vi "Insert View into Subpanel.vi"(0 "GUI Container Actor in":refnum<class "GUI Container Actor.lvclass">, 5 "View":string, 7 "View Hierarchy Level":i32, 9 "Subpanel":string, 11 "error in (no error)":errorcluster) -> (4 "GUI Container Actor out":refnum<class "GUI Container Actor.lvclass">, 15 "error out":errorcluster)   [LabVIEW 2017, in "GUI Views.lvlib" / "GUI Container Actor.lvclass"]
doc: "Inserts the Front Panel of a specified Actor Core VI of the the specified View class hierarchy into a specified subpanel\n\n<b> View </b> String theat contains the name of the View\n\n<b> View Hierarchy Level</b> the level on the subclassing hierarchy of the GUI View actor, it is used to choose the Actor Core Front Panel among all the exisiting sublcasses of the GUI VIew Actor present in the View specified above\n\n<b>Subpanel</b> string designating in which subpanel the Front Panel specified in the above terminals has to be inserted"
uses:
  GUI Container Actor.lvclass
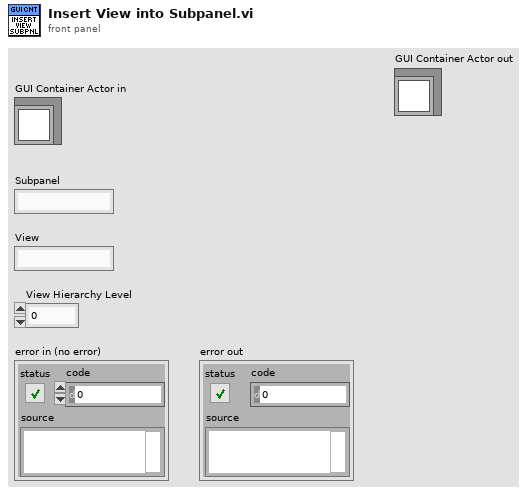
[diagram p1: front panel]
types:
  T1 = typedef "GUI Views.lvlib/GUI Container Actor.lvclass/View Status.ctl" = cluster{"View Details":T2, "Front Panel Statuses":T3[]}
  T2 = typedef "GUI Views.lvlib/GUI Container Actor.lvclass/View Details.ctl" = cluster{"Enqueuer":refnum<class "Message Enqueuer.lvclass">, "VI References":refnum<vi>[], "FP References":refnum<vi>[]}
  T3 = typedef "GUI Views.lvlib/GUI Container Actor.lvclass/FP Status.ctl" = cluster{"FP Open":bool, "Inserted in Subpanel":bool, "Subpanel":string}
  T4 = typedef "GUI Views.lvlib/GUI Container Actor.lvclass/VI References.ctl" = cluster{"FP Ref":refnum<vi>, "VI Ref":refnum<vi>}
  T5 = typedef "GUI Views.lvlib/GUI Container Actor.lvclass/Subpanel Status.ctl" = cluster{"Subpanel Ref":refnum<vi>, "Inserted View":string, "Inserted View Hierarchy Level":i32}
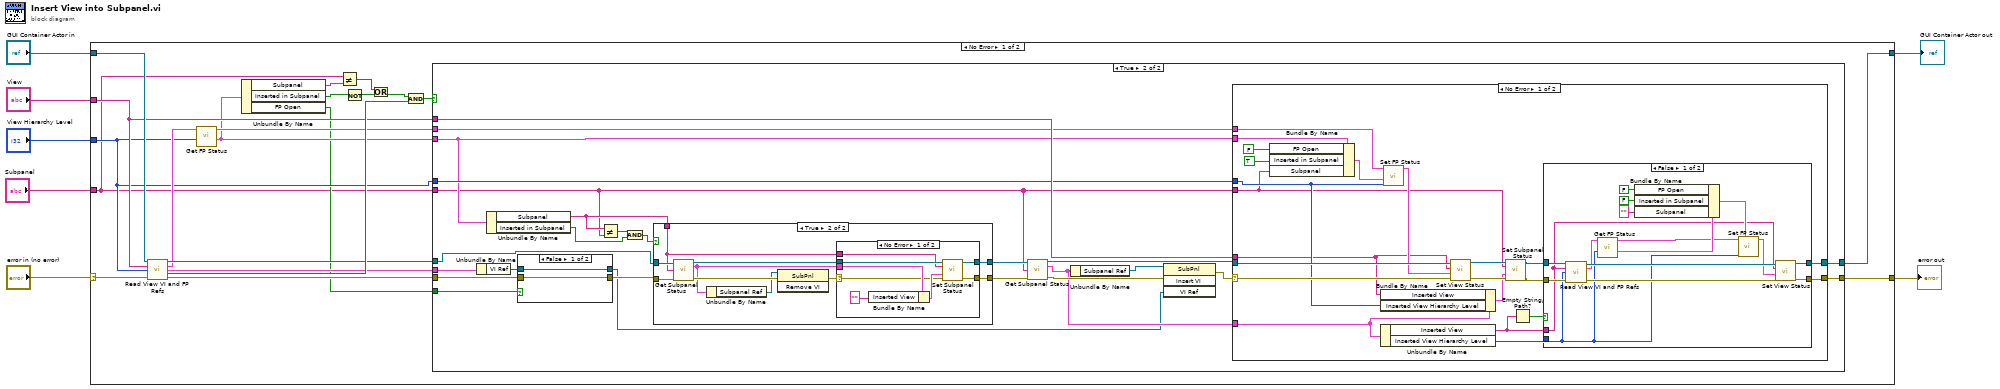
[diagram p0: block diagram]
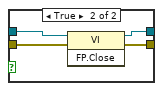
[diagram p7: hidden frame]
diagram:
  n1 = case shown="No Error" "error in (no error)" {
    selector: "error in (no error)" -> [w27 w126]
    tunnel: [w28 w126] -> w7
    tunnel: "GUI Container Actor in" -> [w26 w127]
    tunnel: "Subpanel" -> [w10 _]
    tunnel: "View Hierarchy Level" -> [w15 _]
    tunnel: "View" -> [w20 _]
    tunnel: [w19 w127] -> w1
    frame No Error {
      n2 = call "Read View VI and FP Refs.vi"("GUI Container Actor in"=w26, "View"=w20, "View Hierarchy Level"=w15, "error in (no error)"=w27) -> ("GUI Container Actor out"=w22:refnum<class "GUI Container Actor.lvclass">, "View Status"=w18:T1, "VI References"=w21:T4, "View Found"=w25:bool, "error out"=w23:errorcluster)  [unwired: 7 in]
      n3 = call "Get FP Status.vi"("View Hierarchy Level"=w15, "View Status in"=w18) -> ("FP Status"=w16:T3, "View Status out"=w17:T1)  [unwired: 8 in]
      n4 = Unbundle By Name(w16) -> ("Subpanel"=w13:string, "Inserted in Subpanel"=w11:bool, "FP Open"=w14:bool)
      n5 = Not Equal?(x=w10, y=w13) -> (x != y?=w8:bool)
      n6 = Not(x=w11) -> (.not. x?=w12:bool)
      n7 = Or(x=w8, y=w12) -> (x .or. y?=w9:bool)
      n8 = Compound Arithmetic op=AND(w9, w25) -> (w24:bool)
      n9 = case shown="True" w24 {
        tunnel: [w30 w49] -> w28
        tunnel: w10 -> [_ w31]
        tunnel: w23 -> [w30 w52]
        tunnel: w22 -> [w29 w35]
        tunnel: w21 -> [_ w54]
        tunnel: w14 -> [_ w51]
        tunnel: w20 -> [_ w47]
        tunnel: [w29 w46] -> w19
        tunnel: w17 -> [_ w45]
        tunnel: w16 -> [_ w33]
        tunnel: w15 -> [_ w44]
        frame False {
        }
        frame True {
          n10 = Unbundle By Name(w54) -> ("VI Ref"=w53:refnum<vi>)
          n11 = Unbundle By Name(w33) -> ("Subpanel"=w38:string, "Inserted in Subpanel"=w41:bool)
          n12 = case shown="False" w51 {
            tunnel: w53 -> [w121 w125]
            tunnel: w52 -> [w120 w124]
            tunnel: [w120 w123] -> w36
            tunnel: [w121 w122] -> w32
            frame False {
            }
            frame True {
              n13 = invoke class="VI" method="FP.Close"(reference=w125, error in=w124) -> (reference out=w122:refnum<vi>, error out=w123:errorcluster)  [unwired: 1 in, 1 out]
            }
          }
          n14 = Not Equal?(x=w38, y=w31) -> (x != y?=w39:bool)
          n15 = And(x=w39, y=w41) -> (x .and. y?=w40:bool)
          n16 = case shown="True" w40 {
            tunnel: w36 -> [w56 w67]
            tunnel: w35 -> [w57 w66]
            tunnel: [w57 w64] -> w34
            tunnel: [w56 w63] -> w37
            tunnel: w38 -> [_ w62]
            frame False {
            }
            frame True {
              n17 = call "Get Subpanel Status.vi"("GUI Container Actor in"=w66, "Subpanel"=w62, "error in (no error)"=w67) -> ("GUI Container Actor out"=w65:refnum<class "GUI Container Actor.lvclass">, "Subpanel Status"=w60:T5, "error out"=w61:errorcluster)  [unwired: 9 in, 1 out]
              n18 = Unbundle By Name(w60) -> ("Subpanel Ref"=w59:refnum<vi>)
              n19 = invoke class="SubPnl" method="Remove VI"(reference=w59, error in=w61) -> (error out=w58:errorcluster)  [unwired: 1 in, 2 out]
              n20 = case shown="No Error" w58 {
                selector: w58 -> [w68 w76]
                tunnel: w65 -> [w74 w77]
                tunnel: [w73 w77] -> w64
                tunnel: [w72 w76] -> w63
                tunnel: w62 -> [w70 _]
                tunnel: w60 -> [w69 _]
                frame No Error {
                  n21 = Bundle By Name(cluster=w69, "Inserted View"="") -> (w75:T5)
                  n22 = call "Set Subpanel Status.vi"("GUI Container Actor in"=w74, "Subpanel"=w70, "Subpanel Status"=w75, "error in (no error)"=w68) -> ("GUI Container Actor out"=w73:refnum<class "GUI Container Actor.lvclass">, "error out"=w72:errorcluster)  [unwired: 9 in, 1 out]
                }
                frame Error {
                }
              }
            }
          }
          n23 = call "Get Subpanel Status.vi"("GUI Container Actor in"=w34, "Subpanel"=w31, "error in (no error)"=w37) -> ("GUI Container Actor out"=w48:refnum<class "GUI Container Actor.lvclass">, "Subpanel Status"=w42:T5, "error out"=w55:errorcluster)  [unwired: 9 in, 1 out]
          n24 = Unbundle By Name(w42) -> ("Subpanel Ref"=w43:refnum<vi>)
          n25 = invoke class="SubPnl" method="Insert VI"(reference=w43, error in=w55, "VI Ref"=w32) -> (error out=w50:errorcluster)  [unwired: 1 in, 3 out]
          n26 = case shown="No Error" w50 {
            selector: w50 -> [w98 w119]
            tunnel: [w79 w119] -> w49
            tunnel: w48 -> [w99 w118]
            tunnel: w47 -> [w92 _]
            tunnel: [w80 w118] -> w46
            tunnel: w33 -> [w87 _]
            tunnel: w45 -> [w96 _]
            tunnel: w44 -> [w93 _]
            tunnel: w31 -> [w86 _]
            tunnel: w42 -> [w82 _]
            frame No Error {
              n27 = Bundle By Name(cluster=w87, "FP Open"=FALSE, "Inserted in Subpanel"=TRUE ("FP Open"), "Subpanel"=w86) -> (w89:T3)
              n28 = Unbundle By Name(w82) -> ("Inserted View"=w81:string, "Inserted View Hierarchy Level"=w83:i32)
              n29 = Bundle By Name(cluster=w82, "Inserted View"=w92, "Inserted View Hierarchy Level"=w93) -> (w91:T5)
              n30 = call "Set FP Status.vi"("View Hierarchy Level"=w93, "FP Status"=w89, "View Status in"=w96) -> ("View Status out"=w95:T1)  [unwired: 8 in]
              n31 = call "Set View Status.vi"("error in (no error)"=w98, "View Status"=w95, "View"=w92, "GUI Container Actor in"=w99) -> ("error out"=w94:errorcluster, "GUI Container Actor out"=w90:refnum<class "GUI Container Actor.lvclass">)  [unwired: 5 in, 1 out]
              n32 = call "Set Subpanel Status.vi"("GUI Container Actor in"=w90, "Subpanel"=w86, "Subpanel Status"=w91, "error in (no error)"=w94) -> ("GUI Container Actor out"=w85:refnum<class "GUI Container Actor.lvclass">, "error out"=w84:errorcluster)  [unwired: 9 in, 1 out]
              n33 = Empty String/Path?(string/path=w81) -> (empty?=w78:bool)
              n34 = case shown="False" w78 {
                tunnel: w85 -> [w105 w117]
                tunnel: w84 -> [w104 w116]
                tunnel: w83 -> [w103 _]
                tunnel: w81 -> [w102 _]
                tunnel: [w101 w117] -> w80
                tunnel: [w100 w116] -> w79
                frame False {
                  n35 = call "Read View VI and FP Refs.vi"("GUI Container Actor in"=w105, "View"=w102, "View Hierarchy Level"=w103, "error in (no error)"=w104) -> ("GUI Container Actor out"=w115:refnum<class "GUI Container Actor.lvclass">, "View Status"=w109:T1, "error out"=w114:errorcluster)  [unwired: 7 in, 2 out]
                  n36 = call "Get FP Status.vi"("View Hierarchy Level"=w103, "View Status in"=w109) -> ("FP Status"=w111:T3, "View Status out"=w110:T1)  [unwired: 8 in]
                  n37 = Bundle By Name(cluster=w111, "FP Open"=FALSE, "Inserted in Subpanel"=FALSE, "Subpanel"="") -> (w112:T3)
                  n38 = call "Set FP Status.vi"("View Hierarchy Level"=w103, "FP Status"=w112, "View Status in"=w110) -> ("View Status out"=w113:T1)  [unwired: 8 in]
                  n39 = call "Set View Status.vi"("error in (no error)"=w114, "View Status"=w113, "View"=w102, "GUI Container Actor in"=w115) -> ("error out"=w100:errorcluster, "GUI Container Actor out"=w101:refnum<class "GUI Container Actor.lvclass">)  [unwired: 5 in, 1 out]
                }
                frame True {
                }
              }
            }
            frame Error {
            }
          }
        }
      }
    }
    frame Error {
    }
  }
  "error out" <- w7
  "GUI Container Actor out" <- w1
